vi "TreeSelection Example.vi"() -> ()   [LabVIEW 2015]
doc: "There are three different TreeSelection QControl Classes distributed with the QControl Toolkit. The TreeSelection QControl Class inherits from TreeControl QControl Class.Then the TreeSelectionSingle and TreeSelectionHierarchal QControl Classes inherit from it.\n\nThis example shows how you can extend your own QControls. All three of these classes use the same Event Handler which is found in the parent TreeSelection QControl Class. The extended behavior of the TreeSelectionSingle and TreeSelectionHierarchal QControl Classes are due to the override of some of the methods in TreeSelection QControl Class, namely the ones controlling setup of the checkbox symbols and the toggling rules.\n\n1. Click Run.\n2. Click on the checkboxes in the Trees (click Tab to view others).\n\n a. The tree in the Basic Selection tab will allow any items to be \n selected or deselected.\n b. The tree in the Single Selection tab will allow only one item to be \n selected at a time.\n c. The tree in the Hierarchal Selection tab will control the selection \n given the hierarchy of the tree data.\n\n4. Click Stop to end program.\n\n<b> </b> <b> </b>\n©2016 Q Software Innovations, LLC (QSI)\nwritten by Quentin Alldredge\nproduced in LabVIEW 2015\n\nsupport@qsoftwareinnovations.com\nwww.qsoftwareinnovations.com\n\nAll rights reserved.\n\nRedistribution and use in source and binary forms, with or without modification, are permitted provided that the following conditions are met:\n\n * Redistributions of source code must retain the above copyright notice, this list of conditions and the following disclaimer.\n * Redistributions in binary form must reproduce the above copyright notice, this list of conditions and the following disclaimer in the documentation and/or other materials provided with the distribution.\n * Neither the name of Q Software Innovations, LLC. nor the names of its contributors may be used to endorse or promote products derived from this software without specific prior written permission.\n\nTHIS SOFTWARE IS PROVIDED BY THE COPYRIGHT HOLDERS AND CONTRIBUTORS \"AS IS\" AND ANY EXPRESS OR IMPLIED WARRANTIES, INCLUDING, BUT NOT LIMITED TO, THE IMPLIED WARRANTIES OF MERCHANTABILITY AND FITNESS FOR A PARTICULAR PURPOSE ARE DISCLAIMED. IN NO EVENT SHALL THE COPYRIGHT OWNER OR CONTRIBUTORS BE LIABLE FOR ANY DIRECT, INDIRECT, INCIDENTAL, SPECIAL, EXEMPLARY, OR CONSEQUENTIAL DAMAGES (INCLUDING, BUT NOT LIMITED TO, PROCUREMENT OF SUBSTITUTE GOODS OR SERVICES; LOSS OF USE, DATA, OR PROFITS; OR BUSINESS INTERRUPTION) HOWEVER CAUSED AND ON ANY THEORY OF LIABILITY, WHETHER IN CONTRACT, STRICT LIABILITY, OR TORT (INCLUDING NEGLIGENCE OR OTHERWISE) ARISING IN ANY WAY OUT OF THE USE OF THIS SOFTWARE, EVEN IF ADVISED OF THE POSSIBILITY OF SUCH DAMAGE."
uses:
  QControl Classes/TreeControl/Tree Action Enum.ctl
  QControl Classes/TreeSelection/TreeSelection.lvclass
  QControl Classes/TreeSelectionSingle/TreeSelectionSingle.lvclass
  QControl Classes/TreeSelectionHierarchal/TreeSelectionHierarchal.lvclass
  QControl Classes/TreeControl/TreeControl.lvclass
panel:
  in  "Stop Button":bool
  in  "Tab Control":T1(tab)
  in  "TreeSelection":string(tree)
  in  "TreeSelectionSingle":string(tree)
  in  "TreeSelectionHierarchal":string(tree)
  # "TreeSelection QControl Example\n\nThere are three different TreeSelection QControl Classes distributed with the QControl Toolkit.  The TreeSelection QControl Class inherits from TreeControl QControl Class.Then the TreeSelectionSingle and TreeSelectionHierarchal QControl Classes inherit from it."
  # "This example shows how you can extend your own QControls.  All three of these classes use the same Event Handler which is found in the parent TreeSelection QControl Class.  The extended behavior of the TreeSelectionSingle and TreeSelectionHierarchal QControl Classes are due to the override of some of the methods in TreeSelection QControl Class, namely the ones controlling setup of the checkbox symbols and the toggling rules.\n\n1. Click Run.\n2. Click on the checkboxes in the Trees (click Tab to view others).\n\n  a. The tree in the Basic Selection tab will allow any items to be \n      selected or deselected.\n  b. The tree in the Single Selection tab will allow only one item to be \n      selected at a time.\n  c. The tree in the Hierarchal Selection tab will control the selection \n      given the hierarchy of the tree data.\n\n4. Click Stop to end program."
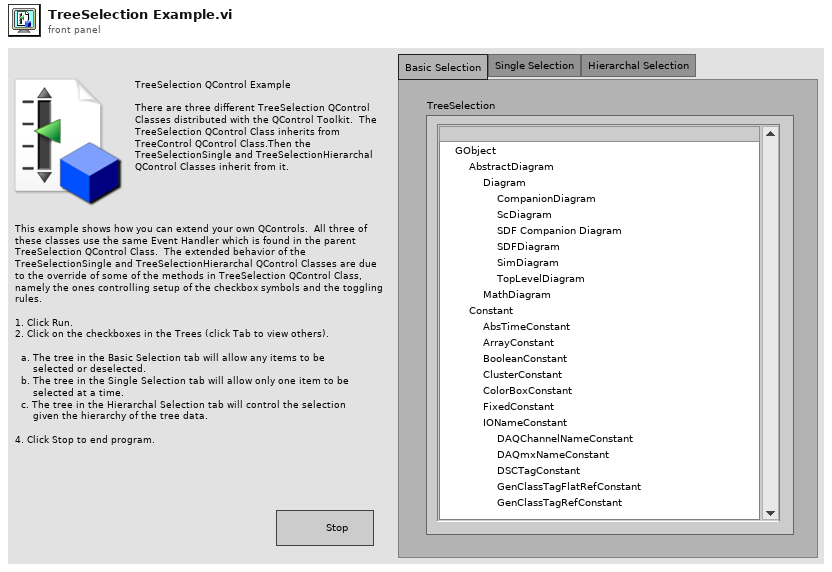
[diagram p1: front panel]
types:
  T1 = enum32{"Basic Selection", "Single Selection", "Hierarchal Selection"}
  T2 = typedef "TreeControl.lvclass/Tree Action Enum.ctl" = enum16{"Open All", "Close All", "Open Item", "Close Item"}
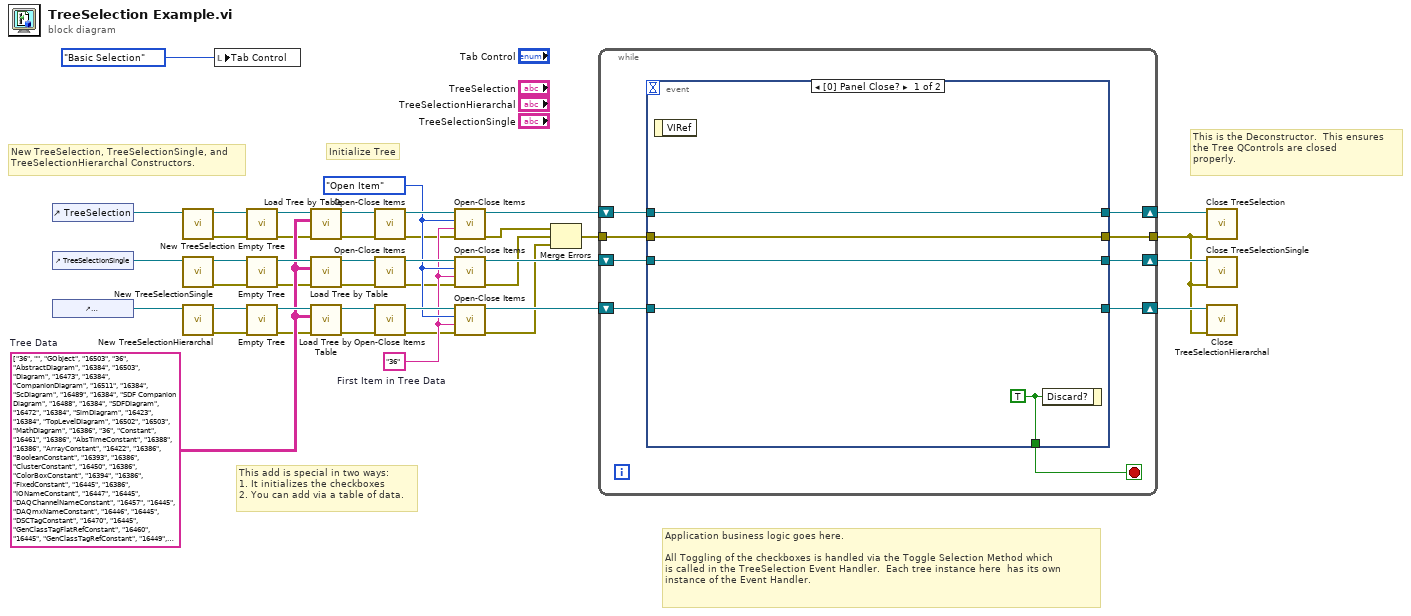
[diagram p0: block diagram]
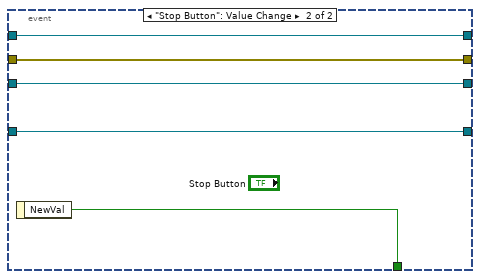
[diagram p2: hidden frame]
diagram:
  w21 = "36"  # First Item in Tree Data
  w22 = Tree_Action_Enum."Open Item" ("Action (Close All)")
  w29 = string[][] [["36", "", "GObject"], ["16503", "36", "AbstractDiagram"], ["16384", "16503", "Diagram"], ["16473", "16384", "CompanionDiagram"], ["16511", "16384", "ScDiagram"], ["16489", "16384", "SDF Companion Diagram"], ["16488", "16384", "SDFDiagram"], ["16472", "16384", "SimDiagram"], ["16423", "16384", "TopLevelDiagram"], ["16502", "16503", "MathDiagram"], ["16386", "36", "Constant"], ["16461", "16386", "AbsTimeConstant"], ["16388", "16386", "ArrayConstant"], ["16422", "16386", "BooleanConstant"], ["16393", "16386", "ClusterConstant"], ["16450", "16386", "ColorBoxConstant"], ["16394", "16386", "FixedConstant"], ["16445", "16386", "IONameConstant"], ["16447", "16445", "DAQChannelNameConstant"], ["16457", "16445", "DAQmxNameConstant"], ["16446", "16445", "DSCTagConstant"], ["16470", "16445", "GenClassTagFlatRefConstant"], ["16460", "16445", "GenClassTagRefConstant"], ["16449", "16445", "IVILogicalNameConstant"], ["16448", "16445", "VISAResourceNameConstant"], ["16501", "16386", "LabVIEWClassConstant"], ["16389", "16386", "NumericConstant"], ["16390", "16389", "DigitalNumericConstant"], ["16391", "16389", "NamedNumericConstant"], ["16425", "16391", "EnumConstant"], ["16424", "16391", "RingConstant"], ["16387", "16386", "PathConstant"], ["16482", "16386", "RefNumConstant"], ["16452", "16482", "ClassSpecifierConstant"], ["16529", "16482", "GenClassRefConst"], ["16538", "16482", "TypedRefNumConstant"], ["16539", "16538", "DataValRefNumConstant"], ["16392", "16386", "StringConstant"], ["16466", "16392", "ComboBoxConstant"], ["6", "36", "Control"], ["60", "6", "AbsTime"], ["16", "6", "ActiveXContainer"], ["14", "6", "Array"], ["8", "6", "Boolean"], ["30", "6", "Cluster"], ["72", "30", "RadioButtonsControl"], ["7", "6", "ColorBox"], ["61", "6", "DigitalTable"], ["22", "6", "GraphChart"], ["25", "22", "IntensityChart"], ["26", "22", "IntensityGraph"], ["92", "22", "MixedSignalGraph"], ["23", "22", "WaveformChart"], ["24", "22", "WaveformGraph"], ["121", "24", "DigitalGraph"], ["83", "24", "XYGraph"], ["28", "6", "IOName"], ["49", "28", "DAQChannelName"], ["57", "28", "DAQmxName"], ["48", "28", "DSCTag"], ["122", "28", "GenClassTagFlatRef"], ["67", "28", "GenClassTagRef"], ["51", "28", "IVILogicalName"], ["50", "28", "VISAResourceName"], ["102", "6", "LabVIEWClassControl"], ["12", "6", "ListBox"], ["10", "6", "LVVariant"], ["127", "6", "MixedCheckbox"], ["46", "6", "MulticolumnListbox"], ["130", "6", "MultiSegmentPipe"], ["17", "6", "Numeric"], ["20", "17", "ColorRamp"], ["18", "17", "Digital"], ["19", "17", "NamedNumeric"], ["35", "19", "Enum"], ["34", "19", "Ring"], ["33", "17", "NumericWithScale"], ["32", "33", "Knob"], ["21", "33", "Slide"], ["53", "6", "PageSelector"], ["55", "53", "TabControl"], ["11", "6", "Path"], ["15", "6", "Picture"], ["78", "6", "Pixmap"], ["70", "6", "PlugInControl"], ["71", "6", "PlugInDDODummyContainer"], ["9", "6", "RefNum"], ["68", "9", "GenClassRef"], ["59", "9", "LVObjectRefNum"], ["58", "59", "VIRefNum"], ["44", "9", "TypedRefNum"], ["135", "44", "DataValRefNum"], ["100", "6", "SceneGraphDisplay"], ["90", "6", "Scrollbar"], ["27", "6", "String"], ["29", "27", "ComboBox"], ["132", "6", "StubDDO"], ["65", "6", "SubPanel"], ["13", "6", "Table"], ["66", "6", "TreeControl"], ["47", "6", "WaveformData"], ["4", "36", "Decoration"], ["5", "4", "Text"], ["39", "5", "NumericText"], ["16459", "36", "FlatSequence"], ["16495", "16459", "TimeFlatSequence"], ["16480", "36", "FlatSequenceInnerTunnel"], ["16481", "36", "FlatSequenceOuterTunnel"], ["16396", "36", "FormulaParameter"], ["16500", "16396", "MathScriptNodeParameter"], ["16464", "16396", "ScriptNodeParameter"], ["16421", "36", "Node"], ["16402", "16421", "CallByRef"], ["16451", "16421", "ControlReferenceConstant"], ["16522", "16421", "FeedbackNode"], ["16409", "16421", "Formula"], ["16504", "16409", "InlineCNode"], ["16499", "16409", "MathScriptNode"], ["16436", "16409", "ScriptNode"], ["16400", "16421", "Function"], ["16437", "16400", "ArrayToCluster"], ["16429", "16400", "Comparison"], ["16535", "16429", "InRangeAndCoerce"], ["16492", "16400", "FileDialog"], ["16432", "16400", "FlattenUnflattenString"], ["16483", "16432", "FlattenString"], ["16433", "16400", "GPIBReadWrite"], ["16430", "16400", "ReadWriteFile"], ["16431", "16400", "TypeCast"], ["16397", "16421", "Global"], ["16410", "16421", "GrowableFunction"], ["16411", "16410", "BuildClusterArray"], ["16476", "16410", "Bundler"], ["16414", "16476", "BuildArray"], ["16415", "16476", "NamedBundler"], ["16417", "16410", "CallLibrary"], ["16416", "16410", "CIN"], ["16412", "16410", "CompoundArithmetic"], ["16438", "16410", "FormatScanString"], ["16413", "16410", "IndexArray"], ["16418", "16410", "ObjectFunction"], ["16505", "16418", "Constructor"], ["16420", "16418", "Invoke"], ["16419", "16418", "Property"], ["16542", "16410", "RegisterForEvents"], ["16477", "16410", "Unbundler"], ["16478", "16477", "NamedUnbundler"], ["16517", "16421", "InPlaceBorderNode"], ["16518", "16517", "InPlaceArrayNode"], ["16530", "16517", "InPlaceArraySplitNode"], ["16519", "16517", "InPlaceClusterNode"], ["16524", "16517", "InPlaceDataValRefNode"], ["16521", "16517", "InPlaceElementNode"], ["16520", "16517", "InPlaceVariantNode"], ["16398", "16421", "Local"], ["16523", "16421", "MathScriptCallByRef"], ["16531", "16421", "SharedVariableDynamicOpen"], ["16532", "16421", "SharedVariableDynamicRead"], ["16533", "16421", "SharedVariableDynamicWrite"], ["16512", "16421", "SharedVariableNode"], ["16465", "16421", "StaticVIReference"], ["16404", "16421", "Structure"], ["16516", "16404", "InPlaceElementStructure"], ["16405", "16404", "Loop"], ["16434", "16405", "ForLoop"], ["16435", "16405", "WhileLoop"], ["16467", "16435", "TimedLoop"], ["16406", "16404", "MultiFrameStructure"], ["16408", "16406", "CaseStructure"], ["16487", "16406", "DisableStructure"], ["16458", "16406", "EventStructure"], ["16407", "16406", "Sequence"], ["16462", "16407", "ExternalNode"], ["16474", "16404", "SimulationNode"], ["16537", "16404", "StatechartStructureNode"], ["16509", "16537", "ForkNode"], ["16510", "16537", "JoinNode"], ["16507", "16537", "JunctionNode"], ["16506", "16537", "RegionNode"], ["16508", "16537", "StateNode"], ["16490", "16404", "SynchronousDataFlowNode"], ["16496", "16404", "TimedSequence"], ["16401", "16421", "SubVI"], ["16526", "16401", "AbstractDynamicDispatch"], ["16528", "16526", "CallParentNode"], ["16527", "16526", "DynamicDispatchSubVI"], ["16453", "16401", "ConfNode"], ["16534", "16401", "GenericSubVI"], ["16443", "16401", "PolymorphicSubVI"], ["16540", "16421", "TextBaseNode"], ["16541", "16540", "ExpressionNode"], ["16403", "16421", "UnitCast"], ["16485", "16421", "XNode"], ["16497", "16485", "XDataNode"], ["75", "36", "Pane"], ["31", "36", "Panel"], ["16484", "36", "PolymorphicVISelector"], ["16444", "36", "PropertyItem"], ["40", "36", "Scale"], ["43", "40", "ColorGraphScale"], ["41", "40", "ColorScale"], ["69", "41", "RotaryColorScale"], ["42", "40", "GraphScale"], ["52", "40", "SlideScale"], ["16428", "36", "SequenceLocal"], ["16475", "36", "SimulationDCO"], ["76", "36", "Splitter"], ["16491", "36", "SynchronousDataFlowDCO"], ["16385", "36", "Terminal"], ["16395", "16385", "ControlTerminal"], ["16441", "16385", "InnerTerminal"], ["16456", "16385", "OuterTerminal"], ["16514", "16385", "ParameterTerminal"], ["16515", "16514", "OverridableParameterTerminal"], ["16493", "36", "TimedStructDCO"], ["16426", "36", "Tunnel"], ["16525", "16426", "ConditionalTunnel"], ["16486", "16525", "SelectorTunnel"], ["16442", "16426", "LeftShiftRegister"], ["16427", "16426", "LoopTunnel"], ["16536", "16426", "RegionTunnel"], ["16399", "16426", "RightShiftRegister"], ["16439", "36", "Wire"]]  # Tree Data
  # "This is the Deconstructor.  This ensures \nthe Tree QControls are closed \nproperly."
  # "Application business logic goes here.\n\nAll Toggling of the checkboxes is handled via the Toggle Selection Method which\nis called in the TreeSelection Event Handler.  Each tree instance here  has its own\ninstance of the Event Handler."
  # "This add is special in two ways:\n1. It initializes the checkboxes\n2. You can add via a table of data."
  # "Initialize Tree"
  # "New TreeSelection, TreeSelectionSingle, and\nTreeSelectionHierarchal Constructors."
  n1 = control-ref of="TreeSelection"() -> (w42:refnum<vi>)
  n2 = control-ref of="TreeSelectionSingle"() -> (w38:refnum<vi>)
  n3 = control-ref of="TreeSelectionHierarchal"() -> (w36:refnum<vi>)
  n4 = call "New TreeSelection.vi"("Reference"=w42) -> ("error out"=w17:errorcluster, "TreeSelection out"=w35:refnum<class "TreeSelection.lvclass">)  [unwired: 9 in]
  n5 = call "New TreeSelectionSingle.vi"("Reference"=w38) -> ("error out"=w13:errorcluster, "TreeSelectionSingle out"=w33:refnum<class "TreeSelectionSingle.lvclass">)  [unwired: 9 in]
  n6 = call "New TreeSelectionHierarchal.vi"("Reference"=w36) -> ("error out"=w9:errorcluster, "TreeSelectionHierarchal out"=w31:refnum<class "TreeSelectionHierarchal.lvclass">)  [unwired: 9 in]
  n7 = local write "Tab Control"(T1."Basic Selection" ("Tab Control")) -> ()
  n8 = call "Empty Tree.vi"("error in (no error)"=w17, "Tree in"=w35) -> ("error out"=w16:errorcluster, "Tree out"=w34:refnum<class "TreeSelection.lvclass">)  [unwired: 8 in]
  n9 = call "Empty Tree.vi"("error in (no error)"=w13, "Tree in"=w33) -> ("error out"=w12:errorcluster, "Tree out"=w32:refnum<class "TreeSelectionSingle.lvclass">)  [unwired: 8 in]
  n10 = call "Empty Tree.vi"("error in (no error)"=w9, "Tree in"=w31) -> ("error out"=w8:errorcluster, "Tree out"=w30:refnum<class "TreeSelectionHierarchal.lvclass">)  [unwired: 8 in]
  n11 = call-dynamic "Load Tree by Table.vi"("error in (no error)"=w16, "Table"=w29, "Tree in"=w34) -> ("error out"=w15:errorcluster, "Tree out"=w28:refnum<class "TreeSelection.lvclass">)  [unwired: 7 in]
  n12 = call-dynamic "Load Tree by Table.vi"("error in (no error)"=w12, "Table"=w29, "Tree in"=w32) -> ("error out"=w11:errorcluster, "Tree out"=w27:refnum<class "TreeSelectionSingle.lvclass">)  [unwired: 7 in]
  n13 = call-dynamic "Load Tree by Table.vi"("error in (no error)"=w8, "Table"=w29, "Tree in"=w30) -> ("error out"=w7:errorcluster, "Tree out"=w26:refnum<class "TreeSelectionHierarchal.lvclass">)  [unwired: 7 in]
  n14 = call-dynamic "Open-Close Items.vi"("error in (no error)"=w15, "Tree in"=w28) -> ("error out"=w14:errorcluster, "Tree out"=w25:refnum<class "TreeSelection.lvclass">)  [unwired: 8 in]
  n15 = call-dynamic "Open-Close Items.vi"("error in (no error)"=w11, "Tree in"=w27) -> ("error out"=w10:errorcluster, "Tree out"=w24:refnum<class "TreeSelectionSingle.lvclass">)  [unwired: 8 in]
  n16 = call-dynamic "Open-Close Items.vi"("error in (no error)"=w7, "Tree in"=w26) -> ("error out"=w6:errorcluster, "Tree out"=w23:refnum<class "TreeSelectionHierarchal.lvclass">)  [unwired: 8 in]
  n17 = call-dynamic "Open-Close Items.vi"("error in (no error)"=w14, "Tag (\"\")"=w21, "Action (Close All)"=w22, "Tree in"=w25) -> ("error out"=w5:errorcluster, "Tree out"=w20:refnum<class "TreeSelection.lvclass">)  [unwired: 6 in]
  n18 = call-dynamic "Open-Close Items.vi"("error in (no error)"=w10, "Tag (\"\")"=w21, "Action (Close All)"=w22, "Tree in"=w24) -> ("error out"=w3:errorcluster, "Tree out"=w19:refnum<class "TreeSelectionSingle.lvclass">)  [unwired: 6 in]
  n19 = call-dynamic "Open-Close Items.vi"("error in (no error)"=w6, "Tag (\"\")"=w21, "Action (Close All)"=w22, "Tree in"=w23) -> ("error out"=w4:errorcluster, "Tree out"=w18:refnum<class "TreeSelectionHierarchal.lvclass">)  [unwired: 6 in]
  n20 = Merge Errors(w5, w3, w4) -> (w2:errorcluster)
  n21 = while {
    shift-right: [w50] -> w41
    shift-left: w18 -> [w51]
    shift-right: [w48] -> w40
    shift-left: w20 -> [w47]
    shift-right: [w46] -> w39
    shift-left: w19 -> [w45]
    tunnel: w2 -> [w43]
    tunnel: [w44] -> w1
    stop <- w49 stop-if-true
    n22 = event shown="[0] Panel Close?" {
      selector: _ -> [_ _]
      dyn-events: _ -> [_ _]
      timeout: _ -> [_ _]
      tunnel: w51 -> [w56 w58]
      tunnel: [w56 w58] -> w50
      tunnel: [w55 w61] -> w49
      tunnel: [w54 w60] -> w48
      tunnel: w47 -> [w54 w60]
      tunnel: [w53 w59] -> w46
      tunnel: w45 -> [w53 w59]
      tunnel: [w52 w57] -> w44
      tunnel: w43 -> [w52 w57]
      event Panel Close? {
        w55 = TRUE ("Discard?")
        n23 = event-data() -> ()  [unwired: 1 in, 1 out]
        n24 = event-data("Discard?"=w55) -> ()  [unwired: 1 in, 1 out]
      }
      event "Stop Button": Value Change {
        n25 = event-data() -> ("NewVal"=w61:bool)  [unwired: 1 in]
      }
    }
  }
  n26 = call "Close TreeSelection.vi"("error in (no error)"=w1, "TreeSelection in"=w40) -> ()  [unwired: 9 in, 1 out]
  n27 = call "Close TreeSelectionSingle.vi"("error in (no error)"=w1, "TreeSelectSingle in"=w39) -> ()  [unwired: 9 in, 1 out]
  n28 = call "Close TreeSelectionHierarchal.vi"("error in (no error)"=w1, "TreeHier in"=w41) -> ()  [unwired: 9 in, 1 out]
